vi "BWC_LEOSerialWriteRead.vi"(4 "Enable Termination\nChar (T)":bool=TRUE, 5 "timeout (10sec)":u32=10000, 7 "error in (no error)":errorcluster, 8 "Perform Two Reads Following Write":bool=TRUE, 9 "Command To Write":string="VER?", 10 "VISA resource name":refnum<visa-resource-name>="COM4") -> (0 "error out":errorcluster, 1 "Ack Resp Bytes":u32, 2 "Completion Response":string, 3 "Acknowledge Response":string)   [LabVIEW 2017]
uses:
  <vilib>/Instr/_visa.llb/VISA Configure Serial Port (Instr).vi
panel:
  out "Completion Resp Bytes":u32
  out "Bytes Written":u32
  in  "Max Read Bytes":u32=80
  in  "flow control (0:none)":u16(ring) items=["None", "XON/XOFF", "RTS/CTS", "XON/XOFF & RTS/CTS", "DTR/DSR", "XON/XOFF & DTR/DSR"]
  in  "stop bits (10: 1 bit)":u16(ring)=10 items=["1.0"=10, "1.5"=15, "2.0"=20]
  in  "baud rate (9600)":u32=9600
  in  "data bits (8)":u16=8 min=5 max=8 step=1
  in  "parity (0:none)":enum16{"None", "Odd", "Even", "Mark", "Space"}(ring)
  in  "termination char\n(0xA = '\\n' = LF)":u8=13 format="%.0x"
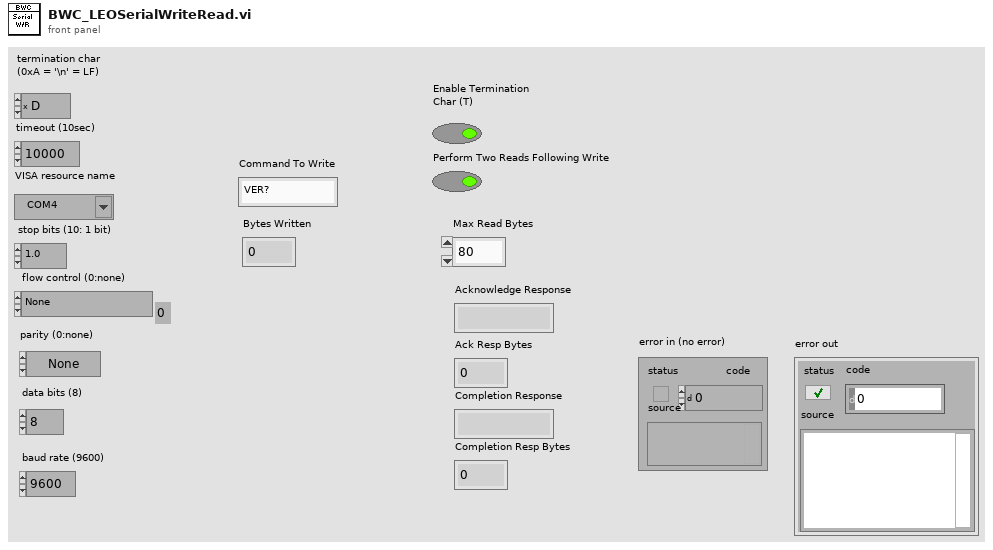
[diagram p1: front panel]
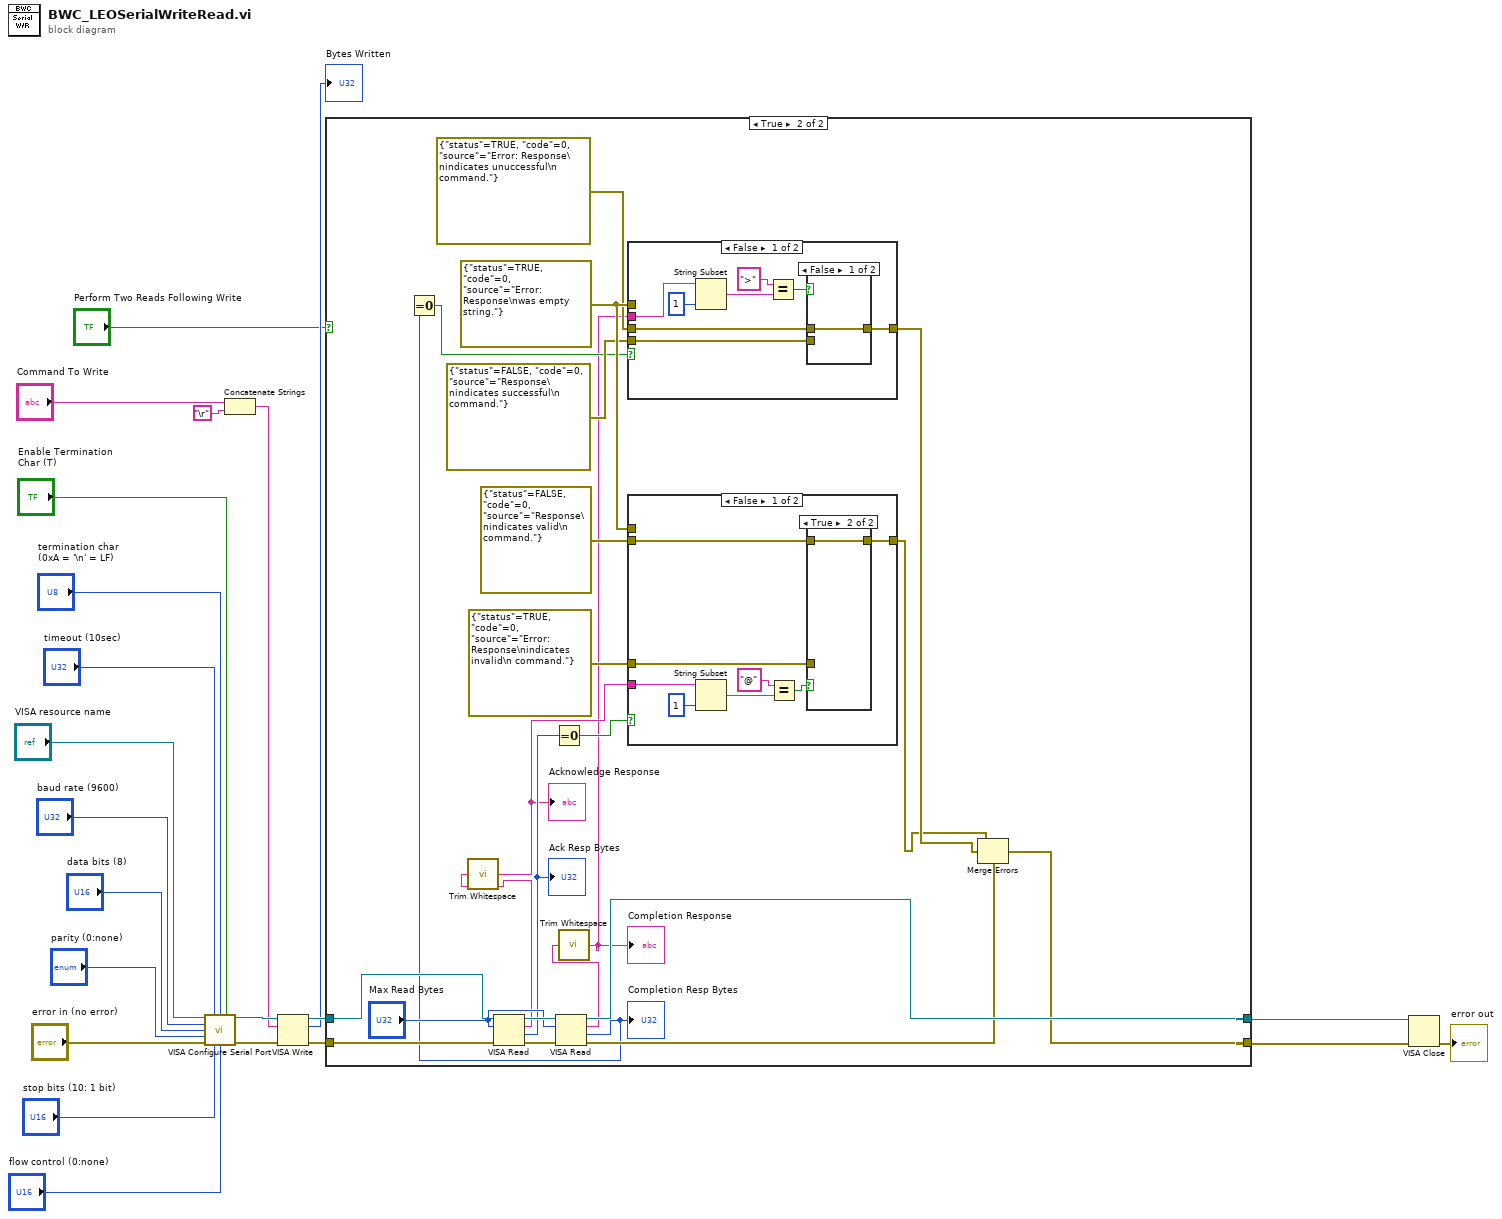
[diagram p0: block diagram]
diagram:
  n1 = call-poly "VISA Configure Serial Port"("VISA resource name"="VISA resource name", "timeout (10sec)"="timeout (10sec)", "termination char\n(0xA = '\\n' = LF)"="termination char\n(0xA = '\\n' = LF)", "Enable Termination\nChar (T)"="Enable Termination\nChar (T)", "baud rate (9600)"="baud rate (9600)", "data bits (8)"="data bits (8)", "parity (0:none)"="parity (0:none)", "error in (no error)"="error in (no error)", "stop bits (10: 1 bit)"="stop bits (10: 1 bit)", "flow control (0:none)"="flow control (0:none)") -> ("VISA resource name out"=w13:refnum<visa-resource-name>, "error out"=w12:errorcluster)  [unwired: 4 in]
  n2 = Concatenate Strings("Command To Write", "\r") -> (w8:string)
  n3 = VISA Write(VISA resource name=w13, write buffer=w8, error in (no error)=w12) -> (VISA resource name out=w6:refnum<visa-resource-name>, return count=→"Bytes Written":u32, error out=w4:errorcluster)
  n4 = case shown="True" "Perform Two Reads Following Write" {
    tunnel: [w24 w42] -> w7
    tunnel: w6 -> [w24 w47]
    tunnel: [w23 w33] -> w5
    tunnel: w4 -> [w23 w46]
    frame False {
    }
    frame True {
      w37 = errorcluster {"status"=TRUE, "code"=0, "source"="Error: Response\nwas empty string."} ("error constant")
      n5 = VISA Read(VISA resource name=w47, byte count="Max Read Bytes", error in (no error)=w46) -> (VISA resource name out=w45:refnum<visa-resource-name>, read buffer=w30:string, return count=w41:u32, error out=w44:errorcluster)
      "Ack Resp Bytes" <- w41
      n6 = call <vilib>:"Trim Whitespace.vi"("string"=w30) -> ("trimmed string"=w29:string)  [unwired: 1 in]
      "Acknowledge Response" <- w29
      n7 = Equal To 0?(x=w41) -> (x = 0?=w40:bool)
      n8 = VISA Read(VISA resource name=w45, byte count="Max Read Bytes", error in (no error)=w44) -> (VISA resource name out=w42:refnum<visa-resource-name>, read buffer=w28:string, return count=w32:u32, error out=w34:errorcluster)
      "Completion Resp Bytes" <- w32
      n9 = Equal To 0?(x=w32) -> (x = 0?=w31:bool)
      n10 = call <vilib>:"Trim Whitespace.vi"("string"=w28) -> ("trimmed string"=w27:string)  [unwired: 1 in]
      "Completion Response" <- w27
      n11 = case shown="False" w31 {
        tunnel: w37 -> [_ w58]
        tunnel: [w50 w58] -> w26
        tunnel: errorcluster {"status"=TRUE, "code"=0, "source"="Error: Response\nindicates unuccessful\n command."} ("error constant") -> [w51 _]
        tunnel: errorcluster {"status"=FALSE, "code"=0, "source"="Response\nindicates successful\n command."} ("error constant") -> [w49 _]
        tunnel: w27 -> [w48 _]
        frame False {
          n12 = String Subset(string=w48, length (rest)=1 ("length (rest)")) -> (substring=w54:string)  [unwired: 1 in]
          n13 = Equal?(x=">", y=w54) -> (x = y?=w52:bool)
          n14 = case shown="False" w52 {
            tunnel: w51 -> [w56 _]
            tunnel: [w56 w57] -> w50
            tunnel: w49 -> [_ w57]
            frame False {
            }
            frame True {
            }
          }
        }
        frame True {
        }
      }
      n15 = case shown="False" w40 {
        tunnel: w37 -> [_ w69]
        tunnel: [w61 w69] -> w25
        tunnel: errorcluster {"status"=TRUE, "code"=0, "source"="Error: Response\nindicates invalid\n command."} ("error constant") -> [w62 _]
        tunnel: errorcluster {"status"=FALSE, "code"=0, "source"="Response\nindicates valid\n command."} ("error constant") -> [w60 _]
        tunnel: w29 -> [w59 _]
        frame False {
          n16 = String Subset(string=w59, length (rest)=1 ("length (rest)")) -> (substring=w65:string)  [unwired: 1 in]
          n17 = Equal?(x="@", y=w65) -> (x = y?=w63:bool)
          n18 = case shown="True" w63 {
            tunnel: w62 -> [w67 _]
            tunnel: [w67 w68] -> w61
            tunnel: w60 -> [_ w68]
            frame False {
            }
            frame True {
            }
          }
        }
        frame True {
        }
      }
      n19 = Merge Errors(w25, w26, w34) -> (w33:errorcluster)
    }
  }
  n20 = VISA Close(VISA resource name=w7, error in (no error)=w5) -> (error out=→"error out":errorcluster)
